vi "VariantClusterToArrayOfValues.vi"(8 "error in (no error)":errorcluster, 11 "Cluster Variant":variant) -> (0 "error out":errorcluster, 1 "Values":variant[](array[variant]), 2 "Names":string[](array[string]))   [LabVIEW 2020]
uses:
  <vilib>/Utility/Data Type/NI_Data Type.lvlib
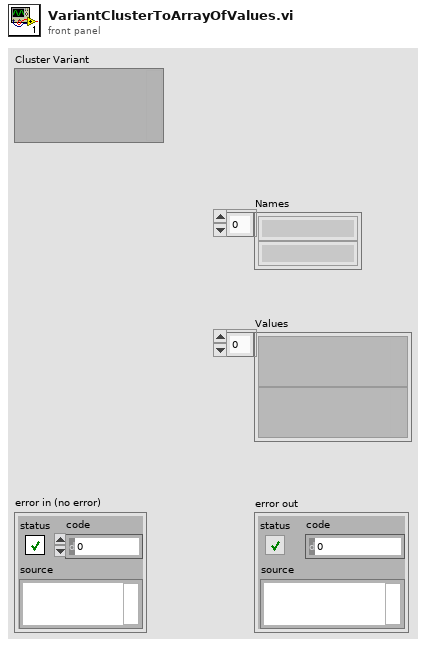
[diagram p1: front panel]
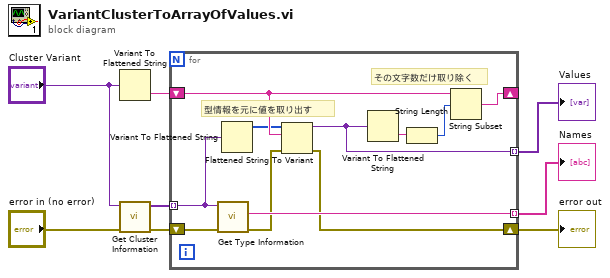
[diagram p0: block diagram]
diagram:
  n1 = Variant To Flattened String(Variant="Cluster Variant") -> (data string=w7:string)  [unwired: 1 out]
  n2 = call <vilib>:"Get Cluster Information.vi"("error in (no error)"="error in (no error)", "variant"="Cluster Variant") -> ("error out"=w3:errorcluster, "cluster elements"=w8:variant[])  [unwired: 8 in]
  n3 = for {
    tunnel: w8 -> [w13] mode=indexing
    shift-right: [w16] -> _
    shift-left: w7 -> [w17]
    tunnel: [w15] -> w6 mode=indexing
    tunnel: [w12] -> w5 mode=indexing
    shift-right: [w10] -> w2
    shift-left: w3 -> [w11]
    # "その文字数だけ取り除く"
    # "型情報を元に値を取り出す"
    n4 = call <vilib>:"Get Type Information.vi"("error in (no error)"=w11, "variant"=w13) -> ("error out"=w9:errorcluster, "name"=w12:string)  [unwired: 5 in, 3 out]
    n5 = Variant To Flattened String(Variant=w13) -> (1:w14:i16[])  [unwired: 1 out]
    n6 = Flattened String To Variant(4:w9, 6:w17, 7:w14) -> (0:w10:errorcluster, 3:w15:variant)
    n7 = Variant To Flattened String(Variant=w15) -> (data string=w19:string)  [unwired: 1 out]
    n8 = String Length(string=w19) -> (length=w18:i32)
    n9 = String Subset(string=w17, offset (0)=w18) -> (substring=w16:string)  [unwired: 1 in]
  }
  "Values" <- w6
  "Names" <- w5
  "error out" <- w2
